vi "getTagEPCBytes.vi"(10 "Data Arry":u8[](array[numeric]) format="%x") -> (2 "EPC Bytes":u8)   [LabVIEW 2018]
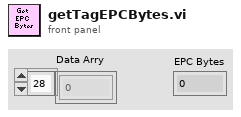
[diagram p1: front panel]
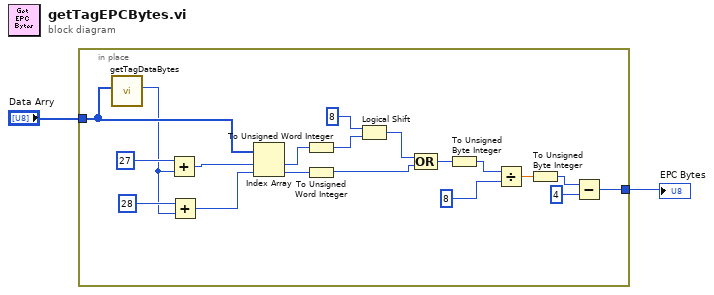
[diagram p0: block diagram]
diagram:
  n1 = in-place {
    in-place-border: "Data Arry" -> [w17]
    in-place-border: [w4] -> w1
    n2 = call "getTagDataBytes.vi"("Data Arry"=w17) -> ("Bytes"=w14:u8)  [unwired: 10 in]
    n3 = Add(x=27 ("index"), y=w14) -> (x+y=w13:i32)
    n4 = Add(x=28 ("index"), y=w14) -> (x+y=w12:i32)
    n5 = Index Array(array=w17, index #1=w13, index #2=w12) -> (element #1=w21:u8, element #2=w20:u8)
    n6 = To Unsigned Word Integer(number=w21) -> (unsigned 16bit integer=w19:u16)
    n7 = To Unsigned Word Integer(number=w20) -> (unsigned 16bit integer=w10:u16)
    n8 = Logical Shift(y=i16 8, x=w19) -> (x << y=w18:u16)
    n9 = Compound Arithmetic op=OR(w18, w10) -> (w9:u16)
    n10 = To Unsigned Byte Integer(number=w9) -> (unsigned 8bit integer=w8:u8)
    n11 = Divide(x=w8, y=u8 8) -> (x/y=w6:dbl)
    n12 = To Unsigned Byte Integer(number=w6) -> (unsigned 8bit integer=w5:u8)
    n13 = Subtract(x=w5, y=u8 4) -> (x-y=w4:u8)
  }
  "EPC Bytes" <- w1
